vi "Revision Query.vi"(8 "error in (no error)":errorcluster, 11 "VISA resource name":refnum<visa-resource-name>) -> (0 "error out":errorcluster, 1 "Instrument Firmware Revision":string, 2 "Instrument Driver Revision":string, 3 "VISA resource name out":refnum<visa-resource-name>)   [LabVIEW 2021, in "BK Precision 9200 Series.lvlib"]
doc: "Queries the current instrument firmware revision and instrument driver revision.\n\nRefer to the Readme file for detailed driver information including modification history."
uses:
  <instrlib>/BK Precision 9200 Series/BK Precision 9200 Series.lvlib
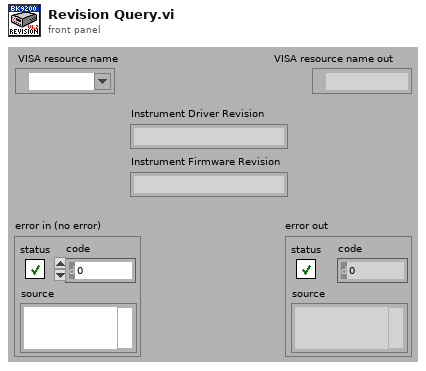
[diagram p1: front panel]
types:
  T1 = cluster{"Major":u16, "Minor":u16, "Fix":u16, "Build":u16}
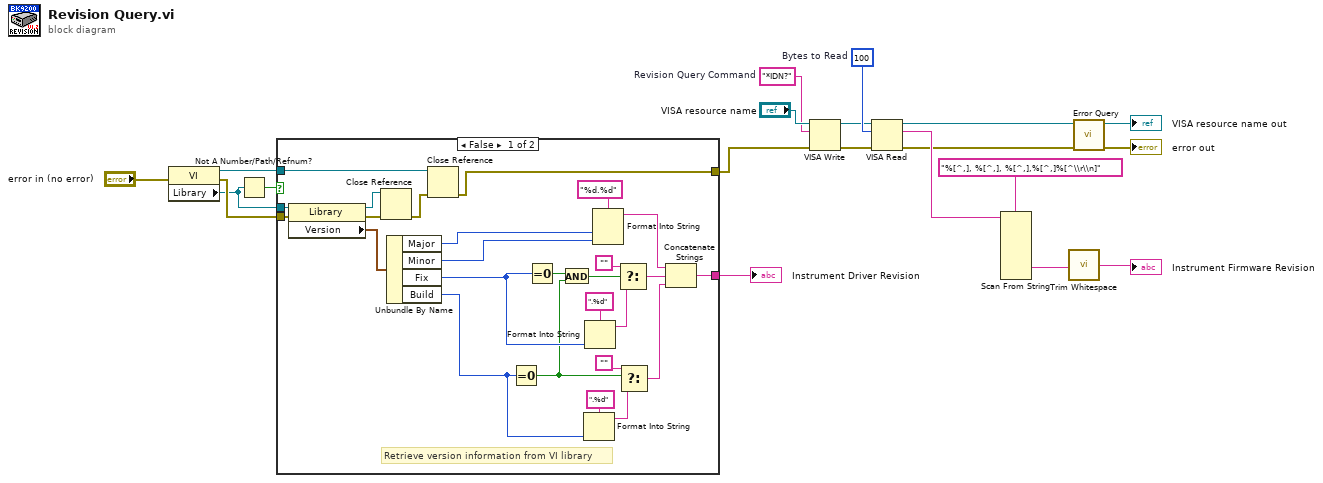
[diagram p0: block diagram]
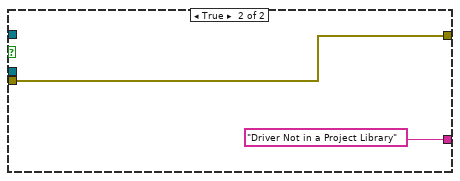
[diagram p2: hidden frame]
diagram:
  w16 = "*IDN?"  # Revision Query Command
  w19 = u32 100  # Bytes to Read
  n1 = property class="VI"(error in="error in (no error)") -> (reference out=w5:refnum<vi>, error out=w4:errorcluster, "Library"=w3:refnum<vi>)  [unwired: 1 in]
  n2 = Not A Number/Path/Refnum?(number/path/refnum=w3) -> (NaN/Path/Refnum?=w2:bool)
  n3 = case shown="False" w2 {
    tunnel: w5 -> [w43 _]
    tunnel: w4 -> [w28 w48]
    tunnel: [w23 w48] -> w8
    tunnel: [w22 "Driver Not in a Project Library"] -> w9
    tunnel: w3 -> [w21 _]
    frame False {
      # "Retrieve version information from VI library"
      n4 = property class="Library"(reference=w21, error in=w28) -> (reference out=w45:refnum<vi>, error out=w46:errorcluster, "Version"=w42:T1)
      n5 = Close Reference(reference=w45, error in (no error)=w46) -> (error out=w44:errorcluster)
      n6 = Unbundle By Name(w42) -> ("Major"=w31:u16, "Minor"=w30:u16, "Fix"=w27:u16, "Build"=w29:u16)
      n7 = Close Reference(reference=w43, error in (no error)=w44) -> (error out=w23:errorcluster)
      n8 = Equal To 0?(x=w29) -> (x = 0?=w25:bool)
      n9 = Equal To 0?(x=w27) -> (x = 0?=w26:bool)
      n10 = And(x=w26, y=w25) -> (x .and. y?=w24:bool)
      n11 = Format Into String(format string=".%d", w29) -> (resulting string=w35:string)  [unwired: 2 in, 1 out]
      n12 = Format Into String(format string=".%d", w27) -> (resulting string=w39:string)  [unwired: 2 in, 1 out]
      n13 = Format Into String(format string="%d.%d", w31, w30) -> (resulting string=w37:string)  [unwired: 2 in, 1 out]
      n14 = Select(t="", s=w24, f=w39) -> (s? t:f=w36:string)
      n15 = Select(t="", s=w25, f=w35) -> (s? t:f=w32:string)
      n16 = Concatenate Strings(w37, w36, w32) -> (w22:string)
    }
    frame True {
    }
  }
  "Instrument Driver Revision" <- w9
  n17 = VISA Write(VISA resource name="VISA resource name", write buffer=w16, error in (no error)=w8) -> (VISA resource name out=w18:refnum<visa-resource-name>, error out=w17:errorcluster)  [unwired: 1 out]
  n18 = VISA Read(VISA resource name=w18, byte count=w19, error in (no error)=w17) -> (VISA resource name out=w12:refnum<visa-resource-name>, read buffer=w15:string, error out=w13:errorcluster)  [unwired: 1 out]
  n19 = Scan From String(format string="%[^,], %[^,], %[^,],%[^,]%[^\\r\\n]", input string=w15) -> (output 4=w7:string)  [unwired: 11 in, 3 out]
  n20 = call <vilib>:"Trim Whitespace.vi"("string"=w7) -> ("trimmed string"=→"Instrument Firmware Revision":string)  [unwired: 1 in]
  n21 = call <instrlib>:"Error Query.vi"("error in (no error)"=w13, "VISA resource name"=w12) -> ("error out"=→"error out":errorcluster, "VISA resource name out"=→"VISA resource name out":refnum<visa-resource-name>)  [unwired: 6 in, 2 out]
